vi "Configure Trigger.vi"(0 "VISA resource name":refnum<visa-resource-name>, 1 "Enable Average Trigger (Disable)":bool, 5 "Measurement Type (6: Phase Noise)":u16(ring)=6 items=["AM Noise"=1, "Baseband Noise"=2, "Freq/Power"=3, "Spectrum"=4, "Transient"=5, "Phase Noise"=6], 7 "Trigger Source (0: Internal)":u16(ring) items=["Internal", "External", "Manual", "Bus", "Wide Video", "Narrow Video"], 9 "Trigger Type (0: Continuous)":u16(ring) items=["Continuous", "Immediate"], 11 "error in (no error)":errorcluster, 12 "External Trigger Polarity (0: Negative)":u16(ring) items=["Negative", "Positive"]) -> (4 "VISA resource name out":refnum<visa-resource-name>, 15 "error out":errorcluster)   [LabVIEW 2011, in "Agilent E5052X.lvlib"]
doc: "Configures trigger settings for any kind of measurement except the User measurement."
uses:
  Agilent E5052X.lvlib
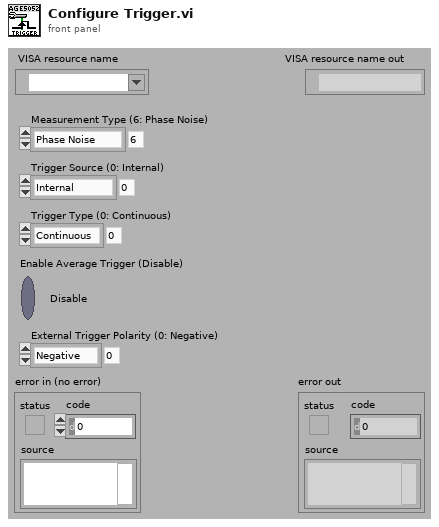
[diagram p1: front panel]
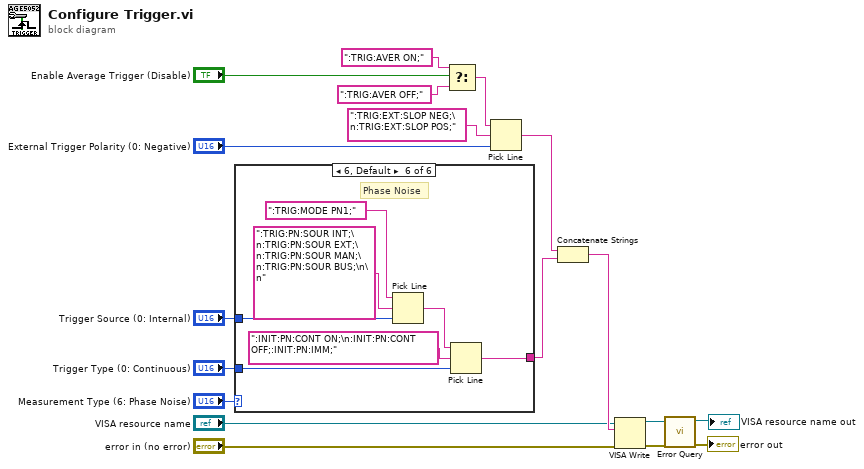
[diagram p0: block diagram]
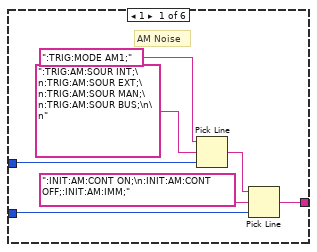
[diagram p2: hidden frame]
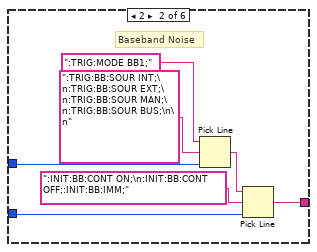
[diagram p3: hidden frame]
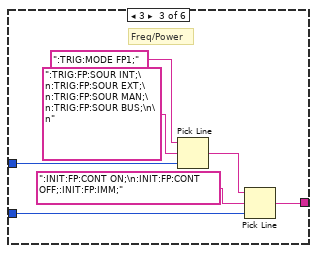
[diagram p4: hidden frame]
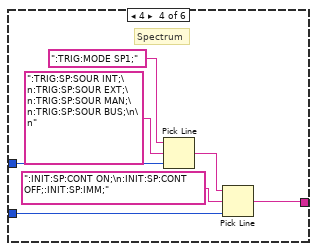
[diagram p5: hidden frame]
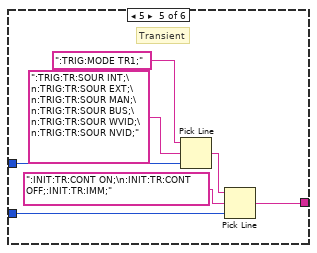
[diagram p6: hidden frame]
diagram:
  n1 = case shown="6, Default" "Measurement Type (6: Phase Noise)" {
    tunnel: "Trigger Source (0: Internal)" -> [w20 w28 w37 w44 w52 w54]
    tunnel: "Trigger Type (0: Continuous)" -> [w19 w27 w35 w42 w48 w56]
    tunnel: [w21 w26 w33 w40 w47 w55] -> w16
    frame 1 {
      # "AM Noise"
      n2 = Pick Line(string ("")=":TRIG:MODE AM1;" ("initial string"), multi-line string=":TRIG:AM:SOUR INT;\n:TRIG:AM:SOUR EXT;\n:TRIG:AM:SOUR MAN;\n:TRIG:AM:SOUR BUS;\n\n", line index=w20) -> (output string=w22:string)
      n3 = Pick Line(string ("")=w22, multi-line string=":INIT:AM:CONT ON;\n:INIT:AM:CONT OFF;:INIT:AM:IMM;", line index=w19) -> (output string=w21:string)
    }
    frame 2 {
      # "Baseband Noise"
      n4 = Pick Line(string ("")=":TRIG:MODE BB1;" ("initial string"), multi-line string=":TRIG:BB:SOUR INT;\n:TRIG:BB:SOUR EXT;\n:TRIG:BB:SOUR MAN;\n:TRIG:BB:SOUR BUS;\n\n", line index=w28) -> (output string=w29:string)
      n5 = Pick Line(string ("")=w29, multi-line string=":INIT:BB:CONT ON;\n:INIT:BB:CONT OFF;:INIT:BB:IMM;", line index=w27) -> (output string=w26:string)
    }
    frame 3 {
      # "Freq/Power"
      n6 = Pick Line(string ("")=":TRIG:MODE FP1;" ("initial string"), multi-line string=":TRIG:FP:SOUR INT;\n:TRIG:FP:SOUR EXT;\n:TRIG:FP:SOUR MAN;\n:TRIG:FP:SOUR BUS;\n\n", line index=w37) -> (output string=w34:string)
      n7 = Pick Line(string ("")=w34, multi-line string=":INIT:FP:CONT ON;\n:INIT:FP:CONT OFF;:INIT:FP:IMM;", line index=w35) -> (output string=w33:string)
    }
    frame 4 {
      # "Spectrum"
      n8 = Pick Line(string ("")=":TRIG:MODE SP1;" ("initial string"), multi-line string=":TRIG:SP:SOUR INT;\n:TRIG:SP:SOUR EXT;\n:TRIG:SP:SOUR MAN;\n:TRIG:SP:SOUR BUS;\n\n", line index=w44) -> (output string=w41:string)
      n9 = Pick Line(string ("")=w41, multi-line string=":INIT:SP:CONT ON;\n:INIT:SP:CONT OFF;:INIT:SP:IMM;", line index=w42) -> (output string=w40:string)
    }
    frame 5 {
      # "Transient"
      n10 = Pick Line(string ("")=":TRIG:MODE TR1;" ("initial string"), multi-line string=":TRIG:TR:SOUR INT;\n:TRIG:TR:SOUR EXT;\n:TRIG:TR:SOUR MAN;\n:TRIG:TR:SOUR BUS;\n:TRIG:TR:SOUR WVID;\n:TRIG:TR:SOUR NVID;", line index=w52) -> (output string=w49:string)
      n11 = Pick Line(string ("")=w49, multi-line string=":INIT:TR:CONT ON;\n:INIT:TR:CONT OFF;:INIT:TR:IMM;", line index=w48) -> (output string=w47:string)
    }
    frame 6, Default {
      # "Phase Noise"
      n12 = Pick Line(string ("")=":TRIG:MODE PN1;" ("initial string"), multi-line string=":TRIG:PN:SOUR INT;\n:TRIG:PN:SOUR EXT;\n:TRIG:PN:SOUR MAN;\n:TRIG:PN:SOUR BUS;\n\n", line index=w54) -> (output string=w57:string)
      n13 = Pick Line(string ("")=w57, multi-line string=":INIT:PN:CONT ON;\n:INIT:PN:CONT OFF;:INIT:PN:IMM;", line index=w56) -> (output string=w55:string)
    }
  }
  n14 = Select(t=":TRIG:AVER ON;", s="Enable Average Trigger (Disable)", f=":TRIG:AVER OFF;") -> (s? t:f=w4:string)
  n15 = Pick Line(string ("")=w4, multi-line string=":TRIG:EXT:SLOP NEG;\n:TRIG:EXT:SLOP POS;", line index="External Trigger Polarity (0: Negative)") -> (output string=w1:string)
  n16 = Concatenate Strings(w1, w16) -> (w15:string)
  n17 = VISA Write(VISA resource name="VISA resource name", write buffer=w15, error in (no error)="error in (no error)") -> (VISA resource name out=w14:refnum<visa-resource-name>, error out=w13:errorcluster)  [unwired: 1 out]
  n18 = call "Error Query.vi"("error in (no error)"=w13, "VISA resource name"=w14) -> ("error out"=→"error out":errorcluster, "VISA resource name out"=→"VISA resource name out":refnum<visa-resource-name>)  [unwired: 6 in, 2 out]
